vi "Parse Successful Login Response.vi"(8 "Error In":errorcluster, 10 "Login Response":string, 11 "Nest Config":T1) -> (0 "Error Out":errorcluster, 3 "Nest Config":T1)   [LabVIEW 2013, in "LMH-Nest.lvlib"]
doc: "Load sesson data from successful login response into Nest config."
uses:
  LMH-Nest.lvlib
  Type Defs/Nest Config.ctl
  <vilib>/httpClient/ClientHandle.ctl
  Type Defs/Session Data.ctl
  <vilib>/express/express shared/NI_ExcelFile/NI_ExcelFile.lvlib
  <vilib>/httpClient/LabVIEWHTTPClient.lvlib
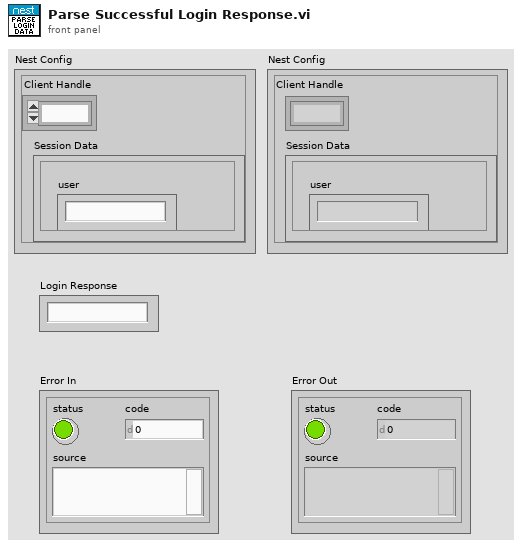
[diagram p1: front panel]
types:
  T1 = typedef "LMH-Nest.lvlib/Nest Config.ctl" = cluster{"Client Handle":T2, "Session Data":T3}
  T2 = typedef "LabVIEWHTTPClient.lvlib/ClientHandle.ctl" = refnum<k1>
  T3 = typedef "LMH-Nest.lvlib/Session Data.ctl" = cluster{"is_superuser":bool, "is_staff":bool, "urls":cluster{"transport_url":string, "rubyapi_url":string, "weather_url":string, "log_upload_url":string, "support_url":string}, "limits":cluster{"thermostats_per_structure":u32, "structures":u32, "thermostats":u32, "smoke_detectors":u32, "smoke_detectors_per_structure":u32}, "access_token":string, "userid":string, "expires_in":string, "email":string, "user":string, "language":string}
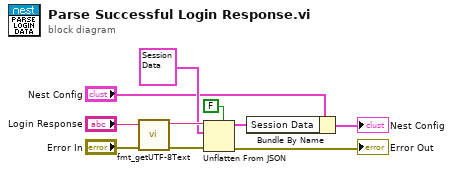
[diagram p0: block diagram]
diagram:
  n1 = call <vilib>:"fmt_getUTF-8Text.vi"("error in"="Error In", "plain text"="Login Response") -> ("error out"=w9:errorcluster, "utf-8 text"=w8:string)  [unwired: 8 in]
  n2 = Unflatten From JSON(enable LabVIEW extensions? (T)=FALSE, JSON string=w8, type and defaults=T3 {"is_superuser"=FALSE, "is_staff"=FALSE, "urls"={"transport_url"="", "rubyapi_url"="", "weather_url"="", "log_upload_url"="", "support_url"=""}, "limits"={"thermostats_per_structure"=0, "structures"=0, "thermostats"=0, "smoke_detectors"=0, "smoke_detectors_per_structure"=0}, "access_token"="", "userid"="", "expires_in"="", "email"="", "user"="", "language"=""} ("Session Data"), error in (no error)=w9) -> (value=w1:T3, error out=→"Error Out":errorcluster)  [unwired: 3 in]
  n3 = Bundle By Name(cluster="Nest Config", "Session Data"=w1) -> (→"Nest Config":T1)
